vi "ReadBackHNSLogs.vi"() -> ()   [LabVIEW 2014]
uses:
  SABL_Source_OLD/HNSCluster.ctl
  SABL_Source_OLD/HNSAI.ctl
  SABL_Source_OLD/HNSWarnings.ctl
  SABL_Source_OLD/HNSMetaCluster.ctl
panel:
  out "Array 2":T1[](array[typedef]) {"Overall Status" format="%x"; "PEP Request Word 2" format="%x"; "PEP Request Word 1" format="%x"}
  out "Numeric 3":i32
  out "Array":T2[](array[typedef])
  out "transposed array":dbl[][](array[numeric])
  out "Numeric 2":i32
  out "Numeric":i32
  out "Waveform Graph":dbl[][](graph)
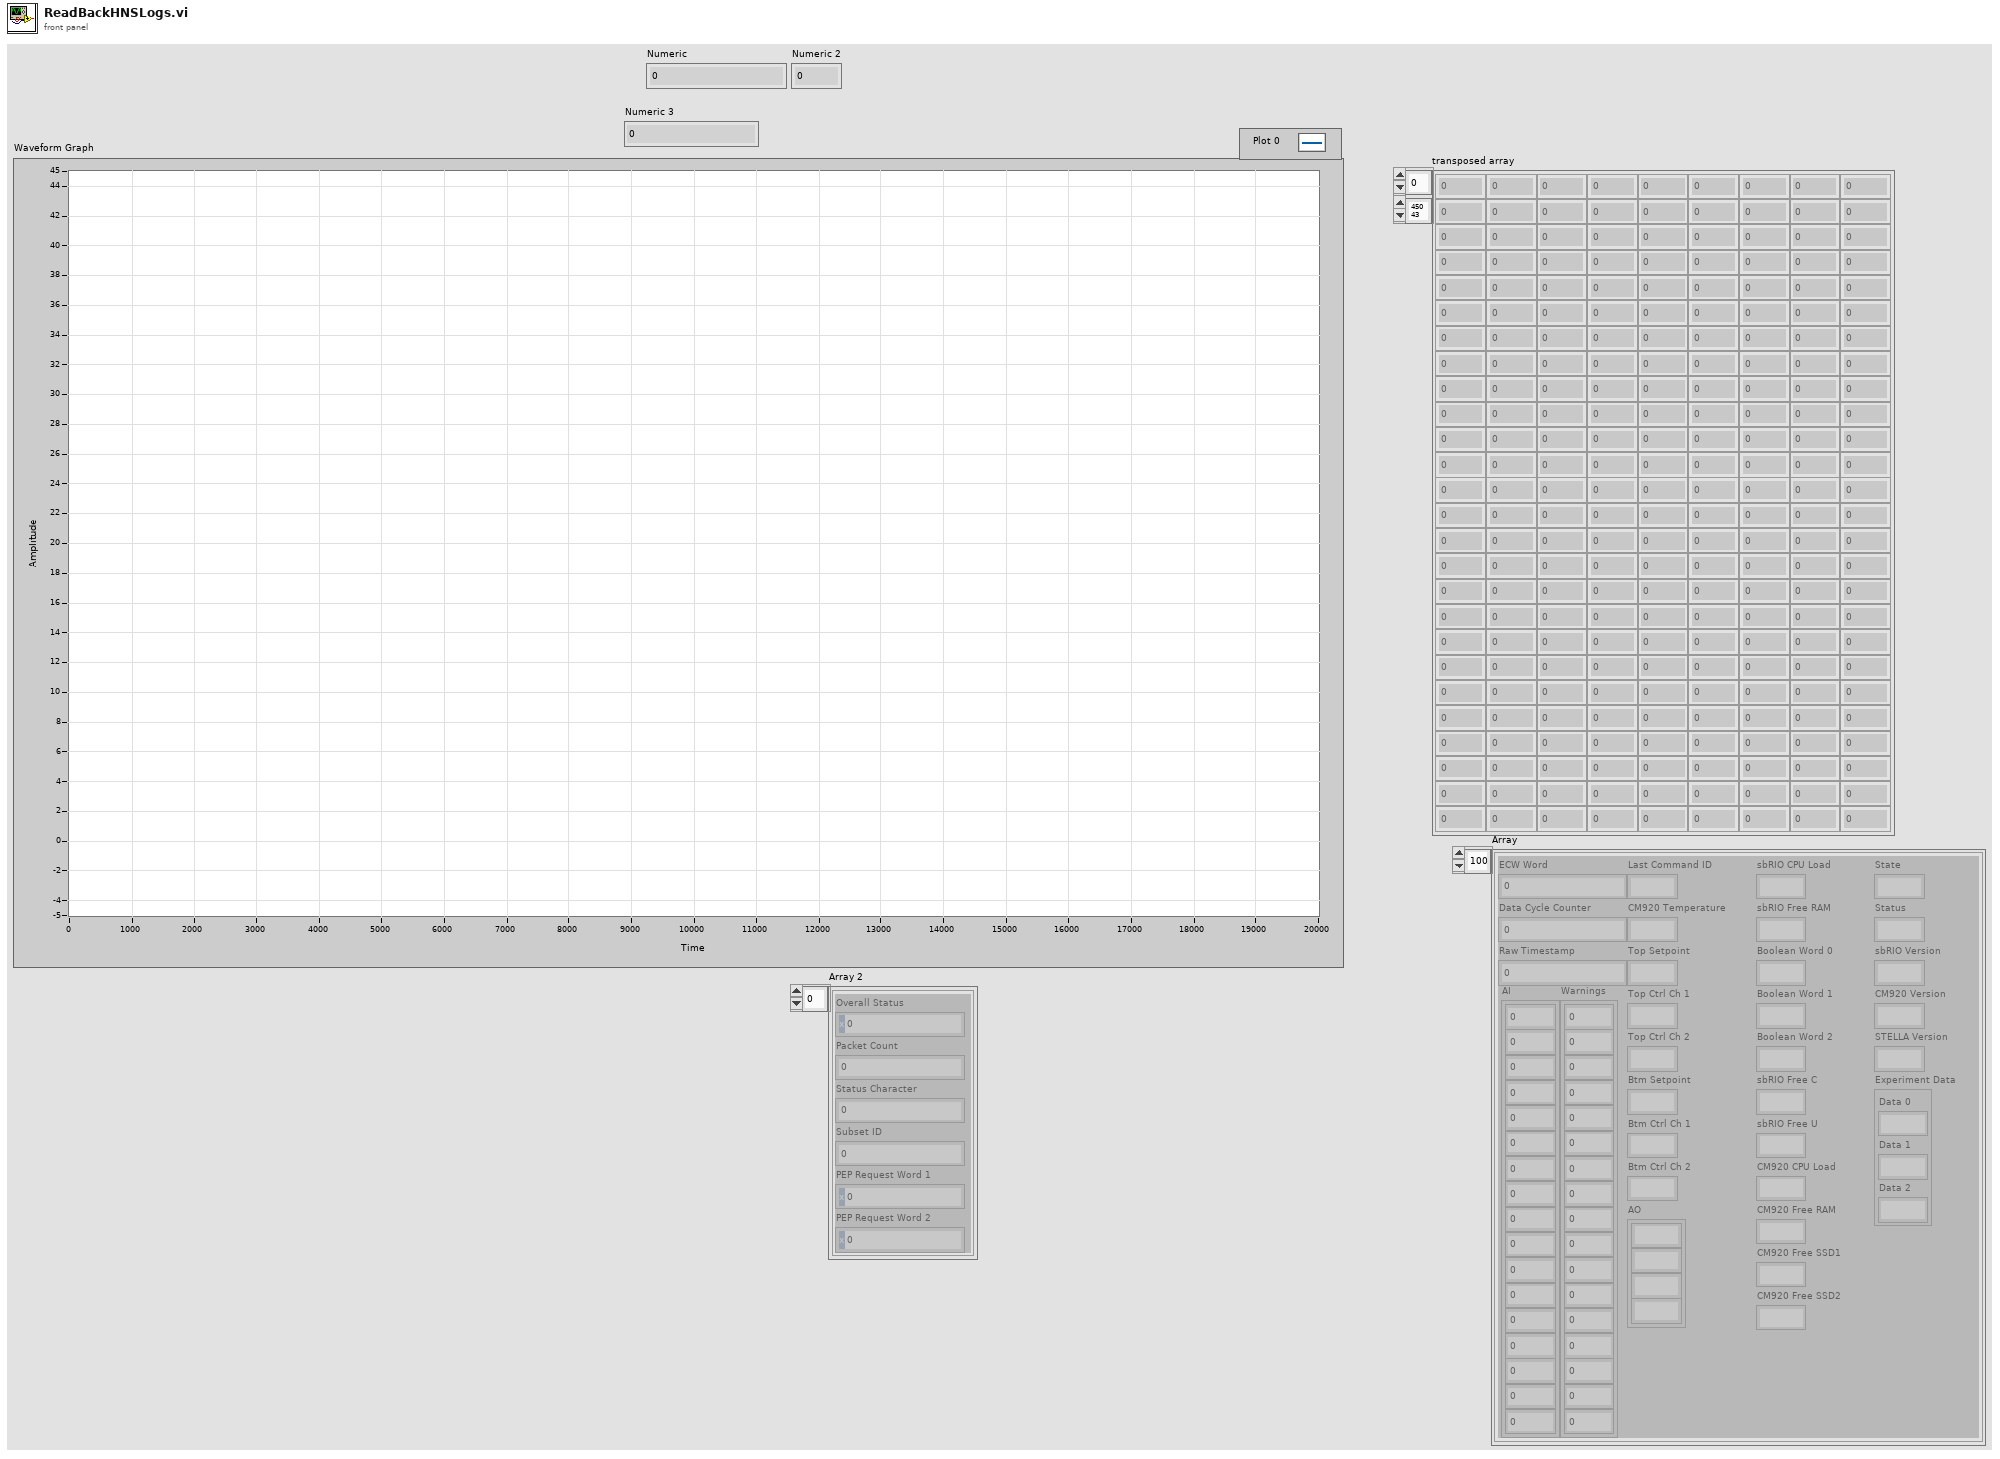
[diagram p1: front panel]
types:
  T1 = typedef "HNSMetaCluster.ctl" = cluster{"Overall Status":u32, "Packet Count":u32, "Status Character":u8, "Subset ID":u16, "PEP Request Word 1":u16, "PEP Request Word 2":u16}
  T2 = typedef "HNSCluster.ctl" = cluster{"ECW Word":u16, "Data Cycle Counter":u16, "Raw Timestamp":dbl, "AI":T3, "Warnings":T4, "Last Command ID":u8, "CM920 Temperature":sgl, "Top Setpoint":sgl, "Top Ctrl Ch 1":i16, "Top Ctrl Ch 2":i16, "Btm Setpoint":sgl, "Btm Ctrl Ch 1":i16, "Btm Ctrl Ch 2":i16, "AO":cluster{sgl, sgl, sgl, sgl}, "sbRIO CPU Load":i16, "sbRIO Free RAM":i16, "Boolean Word 0":i16, "Boolean Word 1":i16, "Boolean Word 2":i16, "sbRIO Free C":i16, "sbRIO Free U":i16, "CM920 CPU Load":i16, "CM920 Free RAM":i16, "CM920 Free SSD1":i16, "CM920 Free SSD2":i16, "State":i16, "Status":i16, "sbRIO Version":sgl, "CM920 Version":sgl, "STELLA Version":sgl, "Experiment Data":cluster{"Data 0":sgl, "Data 1":sgl, "Data 2":sgl}}
  T3 = typedef "HNSAI.ctl" = cluster{"AI0 - Payload Voltage":sgl, "AI1 - Payload Current":sgl, "AI2 - SRM AI1":sgl, "AI3 - SRM AI2":sgl, "AI4 - SRM AI3":sgl, "AI5 - SRM AI4":sgl, "AI6 - Top Back Temp":sgl, "AI7 - Top TEC Current":sgl, "AI8 - Btm Back Temp":sgl, "AI9 - Btm TEC Current":sgl, "AI10 - MTL In Temp":sgl, "AI11 - MTL Out Temp":sgl, "AI12 - Top HX Temp":sgl, "AI13 - Top Front Temp":sgl, "AI14 - Btm HX Temp":sgl, "AI15 - Btm Front Temp":sgl, "AIBT - sbRIO Temp":sgl}
  T4 = typedef "HNSWarnings.ctl" = cluster{"AI0 Warning - Payload Voltage":i8, "AI1 Warning- Payload Current":i8, "AI2 Warning - SRM AI1":i8, "AI3 Warning - SRM AI2":i8, "AI4 Warning - SRM AI3":i8, "AI5 Warning - SRM AI4":i8, "AI6 Warning - Top Back Temp":i8, "AI7 Warning - Top TEC Current":i8, "AI 8 Warning - Btm Back Temp":i8, "AI9 Warning - Btm TEC Current":i8, "AI10 Warning - MTL In Temp":i8, "AI11 Warning - MTL Out Temp":i8, "AI12 Warning - Top HX Temp":i8, "AI13 Warning - Top Front Temp":i8, "AI14 Warning - Btm HX Temp":i8, "AI15 Warning - Btm Front Temp":i8, "AIBT Warning - sbRIO Temp":i8}
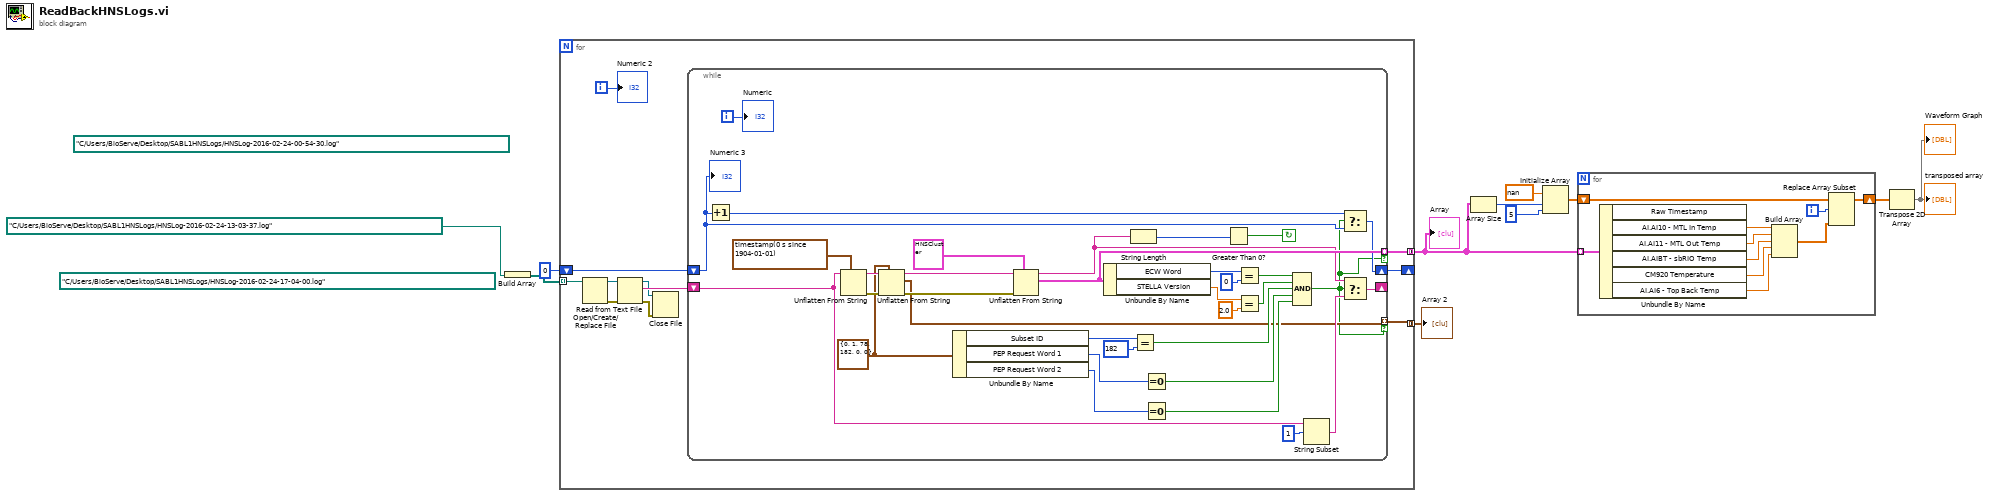
[diagram p0: block diagram]
diagram:
  (unwired) path "C:/Users/BioServe/Desktop/SABL1HNSLogs/HNSLog-2016-02-24-00-54-30.log" ("Folder Path")
  (unwired) path "C:/Users/BioServe/Desktop/SABL1HNSLogs/HNSLog-2016-02-24-17-04-00.log" ("Folder Path")
  n1 = Build Array(path "C:/Users/BioServe/Desktop/SABL1HNSLogs/HNSLog-2016-02-24-13-03-37.log" ("Folder Path")) -> (w3:path[])
  n2 = for {
    tunnel: w3 -> [w22] mode=indexing
    tunnel: [w15] -> w8 mode=concatenating
    shift-right: [w13] -> _
    shift-left: 0 -> [w14]
    tunnel: [w12] -> w1 mode=concatenating
    i -> [w16]
    n3 = Open/Create/Replace File(file path (use dialog)=w22) -> (refnum out=w21:refnum<file>, error out=w20:errorcluster)  [unwired: 5 in, 1 out]
    n4 = Read from Text File(file (use dialog)=w21, error in=w20) -> (refnum out=w17:refnum<file>, text=w19:string, error out=w18:errorcluster)  [unwired: 2 in, 1 out]
    n5 = Close File(refnum=w17, error in=w18) -> ()  [unwired: 2 out]
    n6 = while {
      tunnel: [w49] -> w15 mode=indexing if=w23
      shift-right: [w38] -> _
      shift-left: w19 -> [w40]
      shift-right: [w33] -> w13
      shift-left: w14 -> [w34]
      tunnel: [w24] -> w12 mode=indexing if=w23
      i -> [w54]
      stop <- w36 continue-if-true
      w32 = T1 {"Overall Status"=0, "Packet Count"=1, "Status Character"=78, "Subset ID"=182, "PEP Request Word 1"=0, "PEP Request Word 2"=0} ("HNS Meta Cluster")
      n7 = Increment(x=w34) -> (x+1=w35:i32)
      n8 = Unflatten From String(type=timestamp(0 s since 1904-01-01), binary string=w40) -> (rest of the binary string=w53:string, error out=w50:errorcluster)  [unwired: 3 in, 1 out]
      n9 = Unflatten From String(type=w32, binary string=w53, error in (no error)=w50) -> (rest of the binary string=w52:string, value=w24:T1, error out=w51:errorcluster)  [unwired: 2 in]
      n10 = Unbundle By Name(w32) -> ("Subset ID"=w31:u16, "PEP Request Word 1"=w28:u16, "PEP Request Word 2"=w25:u16)
      n11 = Unflatten From String(type=T2 {"ECW Word"=0, "Data Cycle Counter"=0, "Raw Timestamp"=0.0, "AI"={"AI0 - Payload Voltage"=0.0, "AI1 - Payload Current"=0.0, "AI2 - SRM AI1"=0.0, "AI3 - SRM AI2"=0.0, "AI4 - SRM AI3"=0.0, "AI5 - SRM AI4"=0.0, "AI6 - Top Back Temp"=0.0, "AI7 - Top TEC Current"=0.0, "AI8 - Btm Back Temp"=0.0, "AI9 - Btm TEC Current"=0.0, "AI10 - MTL In Temp"=0.0, "AI11 - MTL Out Temp"=0.0, "AI12 - Top HX Temp"=0.0, "AI13 - Top Front Temp"=0.0, "AI14 - Btm HX Temp"=0.0, "AI15 - Btm Front Temp"=0.0, "AIBT - sbRIO Temp"=0.0}, "Warnings"={"AI0 Warning - Payload Voltage"=0, "AI1 Warning- Payload Current"=0, "AI2 Warning - SRM AI1"=0, "AI3 Warning - SRM AI2"=0, "AI4 Warning - SRM AI3"=0, "AI5 Warning - SRM AI4"=0, "AI6 Warning - Top Back Temp"=0, "AI7 Warning - Top TEC Current"=0, "AI 8 Warning - Btm Back Temp"=0, "AI9 Warning - Btm TEC Current"=0, "AI10 Warning - MTL In Temp"=0, "AI11 Warning - MTL Out Temp"=0, "AI12 Warning - Top HX Temp"=0, "AI13 Warning - Top Front Temp"=0, "AI14 Warning - Btm HX Temp"=0, "AI15 Warning - Btm Front Temp"=0, "AIBT Warning - sbRIO Temp"=0}, "Last Command ID"=0, "CM920 Temperature"=0.0, "Top Setpoint"=0.0, "Top Ctrl Ch 1"=0, "Top Ctrl Ch 2"=0, "Btm Setpoint"=0.0, "Btm Ctrl Ch 1"=0, "Btm Ctrl Ch 2"=0, "AO"={0.0, 0.0, 0.0, 0.0}, "sbRIO CPU Load"=0, "sbRIO Free RAM"=0, "Boolean Word 0"=0, "Boolean Word 1"=0, "Boolean Word 2"=0, "sbRIO Free C"=0, "sbRIO Free U"=0, "CM920 CPU Load"=0, "CM920 Free RAM"=0, "CM920 Free SSD1"=0, "CM920 Free SSD2"=0, "State"=0, "Status"=0, "sbRIO Version"=0.0, "CM920 Version"=0.0, "STELLA Version"=0.0, "Experiment Data"={"Data 0"=0.0, "Data 1"=0.0, "Data 2"=0.0}} ("HNS Cluster"), binary string=w52, error in (no error)=w51) -> (rest of the binary string=w42:string, value=w49:T2)  [unwired: 2 in, 1 out]
      n12 = Unbundle By Name(w49) -> ("ECW Word"=w48:u16, "STELLA Version"=w47:sgl)
      n13 = String Length(string=w42) -> (length=w37:i32)
      n14 = Equal?(x=w31, y=u16 182) -> (x = y?=w29:bool)
      n15 = Equal To 0?(x=w28) -> (x = 0?=w27:bool)
      n16 = Equal To 0?(x=w25) -> (x = 0?=w26:bool)
      n17 = Greater Than 0?(x=w37) -> (x > 0?=w36:bool)
      n18 = Equal?(x=w48, y=u16 0) -> (x = y?=w44:bool)
      n19 = Equal?(x=w47, y=sgl 2.0) -> (x = y?=w43:bool)
      n20 = Compound Arithmetic op=AND(w44, w43, w29, w27, w26) -> (w23:bool)
      n21 = String Subset(string=w40, offset (0)=1) -> (substring=w39:string)  [unwired: 1 in]
      n22 = Select(t=w35, s=w23, f=w34) -> (s? t:f=w33:i32)
      n23 = Select(t=w42, s=w23, f=w39) -> (s? t:f=w38:string)
      "Numeric" <- w54
      "Numeric 3" <- w34
    }
    "Numeric 2" <- w16
  }
  "Array" <- w8
  "Array 2" <- w1
  n24 = Array Size(array=w8) -> (size(s)=w10:i32)
  n25 = Initialize Array(nan, w10, 5 ("dimension size")) -> (w7:dbl[][])
  n26 = for {
    tunnel: w8 -> [w66] mode=indexing
    shift-right: [w57] -> w6
    shift-left: w7 -> [w60]
    i -> [w59]
    n27 = Unbundle By Name(w66) -> ("AI.AI10 - MTL In Temp"=w65:sgl, "AI.AI11 - MTL Out Temp"=w64:sgl, "AI.AIBT - sbRIO Temp"=w63:sgl, "CM920 Temperature"=w62:sgl, "AI.AI6 - Top Back Temp"=w61:sgl)  [unwired: 1 out]
    n28 = Build Array(w65, w64, w63, w62, w61) -> (w58:sgl[])
    n29 = Replace Array Subset(array=w60, new element=w58, index (row)=w59) -> (w57:dbl[][])  [unwired: 1 in]
  }
  n30 = Transpose 2D Array(2D array=w6) -> (transposed array=→"Waveform Graph" →"transposed array":dbl[][])
